vi "Pfeiffer Vacuum Turbo Vent Valve ctrl.vi"(8 "error in (no error)":errorcluster, 9 "PV Vent valve controlling - Cluster":T1={"Parameter"=0, "Parameter\nread only<->describe"=FALSE, "Venting enable\n  off     <-------->     on   "=TRUE, "Venting frequency [%]"=50, "Venting time [s]"=3600, "Venting mode"=0} {"Venting mode" items=[" automatic venting", " do not vent", " venting \"ON\""]; "Venting time [s]" min=6 max=3600 step=1; "Venting frequency [%]" min=40 max=80 step=1; "Parameter" items=[" Venting enable [off / on]", " Venting mode  [0=automatic venting; 1=do not vent; 2=venting \"ON\"]", " Venting frequency  as a % of the final rot. speed of the TMP", " Venting time [s]"]}, 10 "Adress of unit":u16=1 min=1 max=999 step=1, 11 "COM Port Name in":refnum<visa-resource-name>="COM1") -> (0 "error out":errorcluster, 3 "response (data)":string)   [LabVIEW 2016]
doc: "This VI is an example of how to use the Pfeiffer Vacuum subVIs programmatically. This VI first initializes the instrument, takes measurements, then closes the instrument."
uses:
  Public/Turbopumps/PV Ventig time - Cluster.ctl
  Pfeiffer Vacuum.lvlib
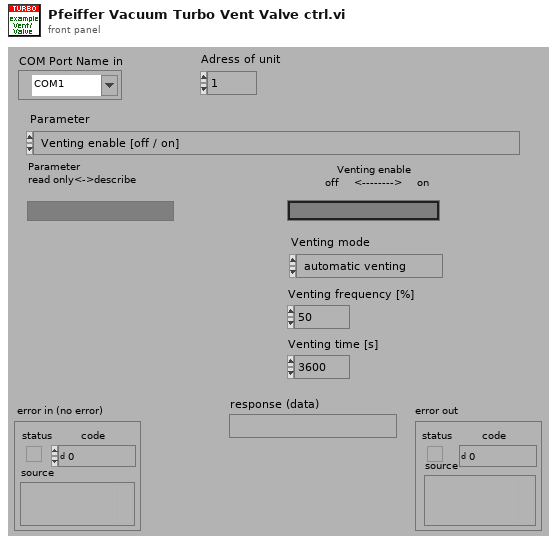
[diagram p1: front panel]
types:
  T1 = typedef "Pfeiffer Vacuum.lvlib/PV Ventig time - Cluster.ctl" = cluster{"Parameter":u16, "Parameter\nread only<->describe":bool, "Venting enable\n  off     <-------->     on   ":bool, "Venting frequency [%]":u16, "Venting time [s]":u16, "Venting mode":u16}
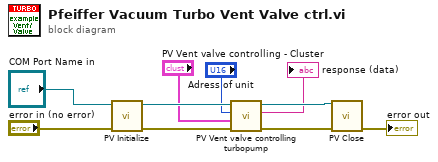
[diagram p0: block diagram]
diagram:
  n1 = call "PV Initialize.vi"("error in (no error)"="error in (no error)", "VISA session in"="COM Port Name in") -> ("error out"=w10:errorcluster, "VISA session out"=w8:refnum<visa-resource-name>)  [unwired: 8 in]
  n2 = call "PV Vent valve controlling turbopump.vi"("error in (no error)"=w10, "PV Vent valve controlling - Cluster"="PV Vent valve controlling - Cluster", "Adress of unit"="Adress of unit", "VISA session"=w8) -> ("error out"=w9:errorcluster, "response (data)"=→"response (data)":string, "dup VISA session"=w7:refnum<visa-resource-name>)  [unwired: 5 in]
  n3 = call "PV Close.vi"("VISA session"=w7, "error in (no error)"=w9) -> ("error out"=→"error out":errorcluster)  [unwired: 13 in]
